vi "Set Temperature.vi"(8 "error in (no error)":errorcluster, 10 "Setpoint":dbl, 11 "Julabo Fp-50 Settings":T1={"VISA resource name"="", "Simulated?"=FALSE, "Pump Power"=2} {"Pump Power" min=0 max=8 step=1}) -> (0 "error out":errorcluster, 1 "Connection Error":bool, 3 "Julabo FP-50 Settings":T1={"VISA resource name"="", "Simulated?"=FALSE, "Pump Power"=2} {"Pump Power" min=0 max=8 step=1})   [LabVIEW 2018, in "Julabo Type FP-50 TCU.lvlib"]
uses:
  Julabo Type FP-50 TCU.lvlib
  Julabo FP-50 Settings.ctl
  Third Party Drivers/Julabo Type 1/JULABO DeviceDriver/JULABO DeviceDriver.lvlib
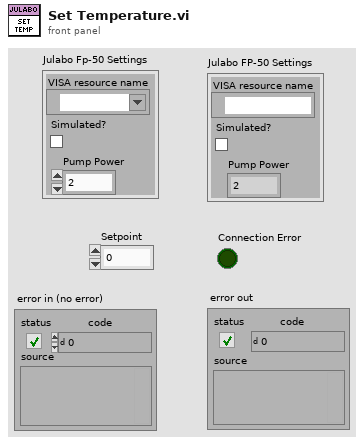
[diagram p1: front panel]
types:
  T1 = typedef "Julabo Type FP-50 TCU.lvlib/Julabo FP-50 Settings.ctl" = cluster{"VISA resource name":refnum<visa-resource-name>, "Simulated?":bool, "Pump Power":i32}
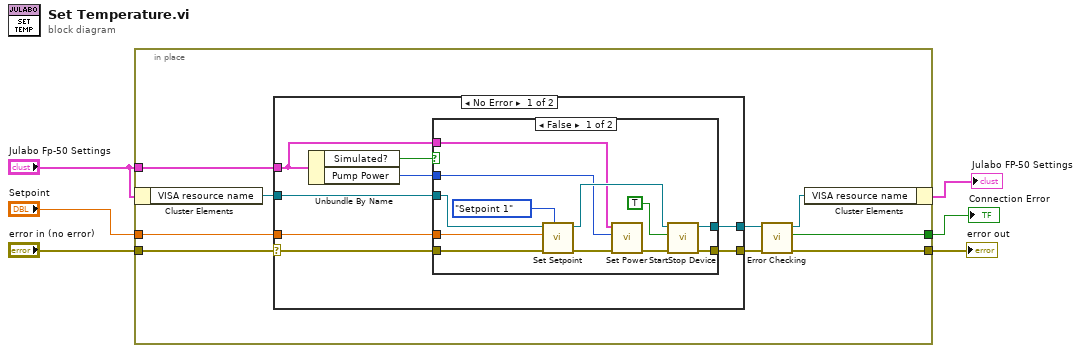
[diagram p0: block diagram]
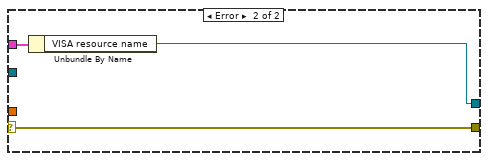
[diagram p3: hidden frame]
diagram:
  n1 = in-place {
    in-place-border: "error in (no error)" -> [w15]
    in-place-border: [w12] -> w5
    in-place-border: "Julabo Fp-50 Settings" -> [w11]
    in-place-border: [w10] -> w4
    in-place-border: "Setpoint" -> [w7]
    n2 = in-place-cluster #1("Julabo Fp-50 Settings") -> ("VISA resource name"=w9:refnum<visa-resource-name>)
    n3 = case shown="No Error" w15 {
      selector: w15 -> [w23 w40]
      tunnel: w11 -> [w19 w39]
      tunnel: [w22 w40] -> w13
      tunnel: [w21 w38] -> w14
      tunnel: w9 -> [w17 _]
      tunnel: w7 -> [w16 _]
      frame No Error {
        n4 = Unbundle By Name(w19) -> ("Simulated?"=w20:bool, "Pump Power"=w18:i32)
        n5 = case shown="False" w20 {
          tunnel: w23 -> [w30 w37]
          tunnel: [w24 w37] -> w22
          tunnel: [w29 w36] -> w21
          tunnel: w17 -> [w32 w36]
          tunnel: w19 -> [w28 _]
          tunnel: w16 -> [w35 _]
          tunnel: w18 -> [w27 _]
          frame False {
            n6 = call "Set Setpoint.vi"("Setpointindex (Setpoint1: Default)"=enum16{"Setpoint 1", "Setpoint 2", "Setpoint 3"}."Setpoint 1", "error in (no error)"=w30, "newSetpoint (20.00°C)"=w35, "VISA resource name"=w32) -> ("error out"=w26:errorcluster, "VISA resource name out"=w31:refnum<visa-resource-name>)  [unwired: 6 in]
            n7 = call "Set Power.vi"("error in (no error)"=w26, "Power"=w27, "Julabo FP-50 Settings"=w28) -> ("error out"=w25:errorcluster)  [unwired: 6 in, 2 out]
            n8 = call "StartStop Device.vi"("error in (no error)"=w25, "Start/Stop (f:Stop)"=TRUE, "VISA resource name"=w31) -> ("error out"=w24:errorcluster, "VISA resource name out"=w29:refnum<visa-resource-name>)  [unwired: 7 in]
          }
          frame True {
          }
        }
      }
      frame Error {
        n9 = Unbundle By Name(w39) -> ("VISA resource name"=w38:refnum<visa-resource-name>)
      }
    }
    n10 = call "Error Checking.vi"("error in (no error)"=w13, "VISA resource name"=w14) -> ("error out"=w12:errorcluster, "Connection Error"=w10:bool, "VISA resource name"=w8:refnum<visa-resource-name>)  [unwired: 7 in]
    n11 = in-place-cluster #1("VISA resource name"=w8) -> (→"Julabo FP-50 Settings":T1)
  }
  "error out" <- w5
  "Connection Error" <- w4
